vi "CreateMutateIcon.vi"(8 "error in (no error)":errorcluster, 10 "New BlueSerializableVersion":u16, 11 "Icon.lvclass in":refnum<class "Icon.lvclass">) -> (0 "error out":errorcluster, 2 "Picture":picture, 3 "Icon.lvlclass out":refnum<class "Icon.lvclass">)   [LabVIEW 2019, in "BlueSerializationScripts.lvlib"]
uses:
  BlueSerializationScripts.lvlib
  <vilib>/LabVIEW Icon API/lv_icon/Classes/Icon/Icon.lvclass
  <vilib>/LabVIEW Icon API/API_Text.ctl
  <vilib>/LabVIEW Icon API/API_Test Settings.ctl
  <vilib>/LabVIEW Icon API/lv_icon/Controls/Alignment.ctl
  <vilib>/LabVIEW Icon API/API_Text Colors.ctl
  <vilib>/LabVIEW Icon API/LabVIEW Icon API.lvlib
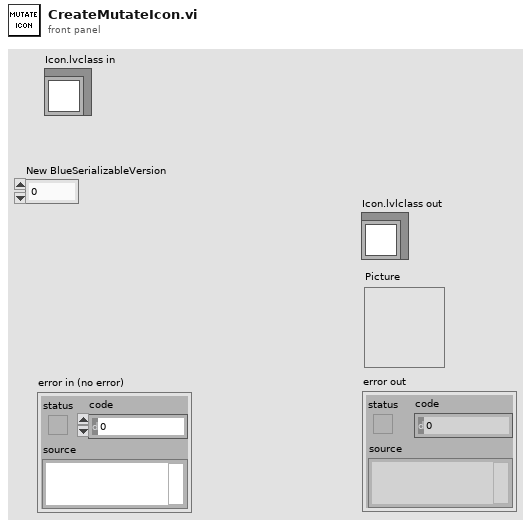
[diagram p1: front panel]
types:
  T1 = typedef "LabVIEW Icon API.lvlib/API_Test Settings.ctl" = cluster{"Font":string, "Alignment":T2, "Size":u8, "Center text":bool, "Capitalize text":bool, "Text color":T3}
  T2 = typedef "Alignment.ctl" = u16
  T3 = typedef "LabVIEW Icon API.lvlib/API_Text Colors.ctl" = cluster{"Line 1 color":u32, "Line 2 color":u32, "Line 3 color":u32, "Line 4 color":u32}
  T4 = typedef "LabVIEW Icon API.lvlib/API_Text.ctl" = cluster{"Line 1 text":string, "Line 2 text":string, "Line 3 text":string, "Line 4 text":string}
  T5 = typedef "imagedata.ctl" = cluster{"image type":i32, "image depth":i32, "image":u8[], "mask":u8[], "colors":u32[], "Rectangle":cluster{"left":i16, "top":i16, "right":i16, "bottom":i16}}
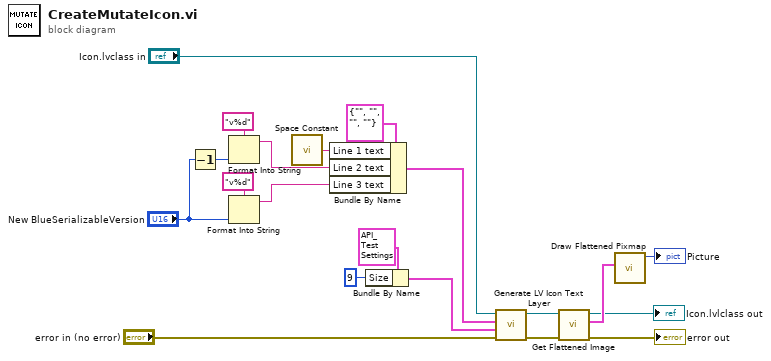
[diagram p0: block diagram]
diagram:
  n1 = Decrement(x="New BlueSerializableVersion") -> (x-1=w4:u16)
  n2 = Format Into String(format string="v%d", w4) -> (resulting string=w5:string)  [unwired: 2 in, 1 out]
  n3 = Format Into String(format string="v%d", "New BlueSerializableVersion") -> (resulting string=w1:string)  [unwired: 2 in, 1 out]
  n4 = call <vilib>:"Space Constant.vi"() -> ("String"=w2:string)
  n5 = Bundle By Name(cluster=T4 {"Line 1 text"="", "Line 2 text"="", "Line 3 text"="", "Line 4 text"=""} ("Text"), "Line 1 text"=w2, "Line 2 text"=w5, "Line 3 text"=w1) -> (w15:T4)
  n6 = Bundle By Name(cluster=T1 {"Font"="Small Fonts", "Alignment"=1, "Size"=8, "Center text"=TRUE, "Capitalize text"=TRUE, "Text color"={"Line 1 color"=0, "Line 2 color"=0, "Line 3 color"=0, "Line 4 color"=0}} ("Text settings"), "Size"=u8 9) -> (w12:T1)
  n7 = call <vilib>:"Generate LV Icon Text Layer.vi"("error in (no error)"="error in (no error)", "Text settings"=w12, "Text"=w15, "Icon in"="Icon.lvclass in") -> ("error out"=w10:errorcluster, "Icon out"=w11:refnum<class "Icon.lvclass">)  [unwired: 6 in]
  n8 = call <vilib>:"Get Flattened Image.vi"("error in (no error)"=w10, "lv_icon.lvlib:Icon.lvclass in"=w11) -> ("error out"=→"error out":errorcluster, "Color Image"=w20:T5, "lv_icon.lvlib:Icon.lvclass out"=→"Icon.lvlclass out":refnum<class "Icon.lvclass">)  [unwired: 6 in, 1 out]
  n9 = call <vilib>:"Draw Flattened Pixmap.vi"("image data"=w20) -> ("new picture"=→"Picture":picture)  [unwired: 8 in]
